vi "ReadProjectSelect.vi"(8 "error in (no error)":errorcluster, 11 "Project.lvclass In":refnum<class "Project.lvclass">) -> (0 "error out":errorcluster, 2 "ProjectSelectIdx":i32, 3 "Project.lvclass Out":refnum<class "Project.lvclass">)   [LabVIEW 2014, in "Project.lvclass"]
uses:
  Project.lvclass
  Project.lvclass/Project.ctl
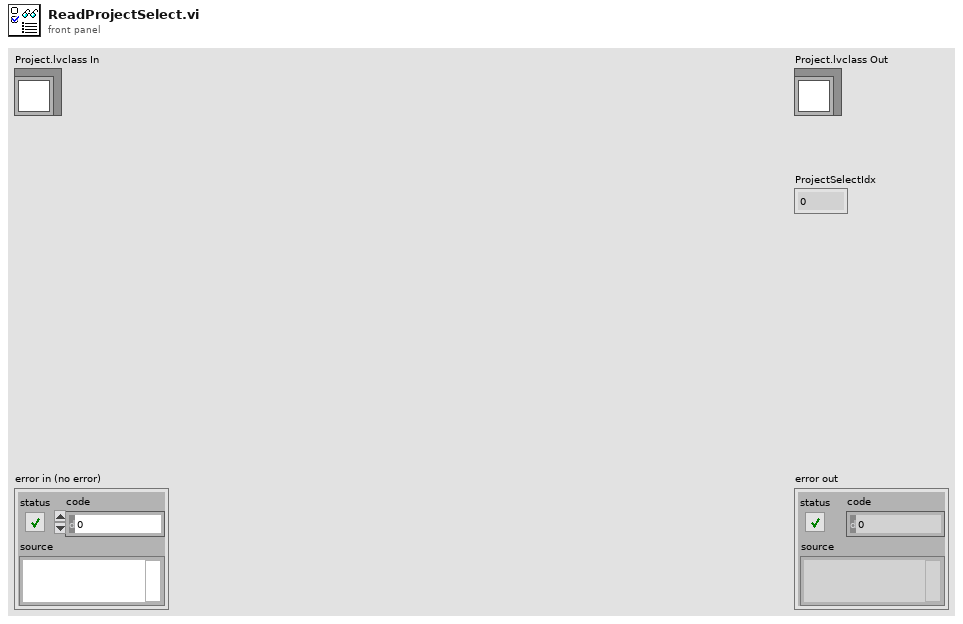
[diagram p1: front panel]
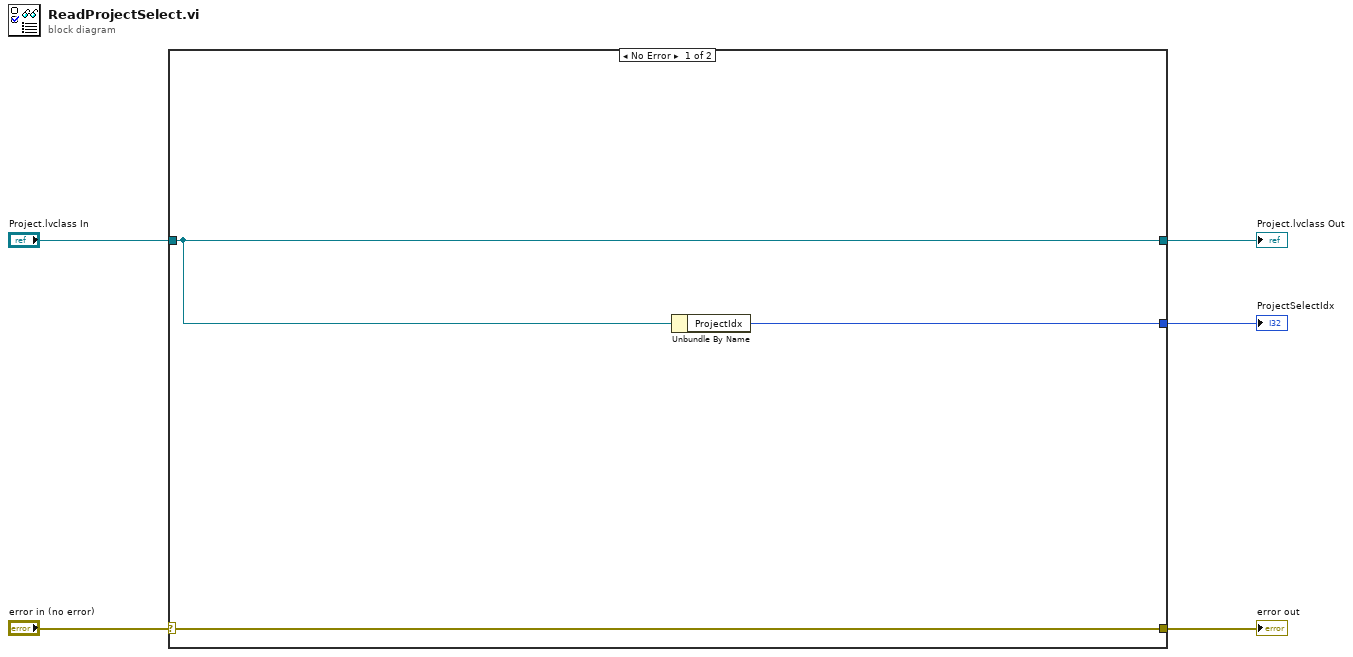
[diagram p0: block diagram]
diagram:
  n1 = case shown="No Error" "error in (no error)" {
    selector: "error in (no error)" -> [w8 w10]
    tunnel: [w8 w10] -> w4
    tunnel: "Project.lvclass In" -> [w7 w9]
    tunnel: [w7 w9] -> w2
    tunnel: [w6 _] -> w1
    frame No Error {
      n2 = Unbundle By Name(w7) -> ("ProjectIdx"=w6:i32)
    }
    frame Error {
    }
  }
  "error out" <- w4
  "Project.lvclass Out" <- w2
  "ProjectSelectIdx" <- w1
